vi "init_img_Q.vi"(2 "max queue size (-1, unlimited)":i32) -> (8 "Image Q Out":T1)   [LabVIEW 2023]
uses:
  <vilib>/vision/Image Controls.llb/IMAQ Image.ctl
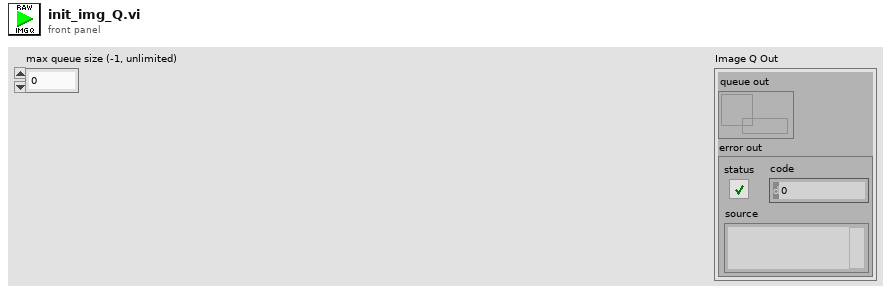
[diagram p1: front panel]
types:
  T1 = cluster{"queue out":refnum<queue>, "error out":errorcluster}
  T2 = typedef "IMAQ Image.ctl" = refnum<image>
  T3 = cluster{"Image Out":T2, "Image Data":cluster{"Actual Width":u32, "Actual Height":u32, "Buffer Number":i32}, "Imaging Variables In":cluster{"Region of interest":i32[], "Number of buffers":u32, "Frame timeout (ms)":u32}}
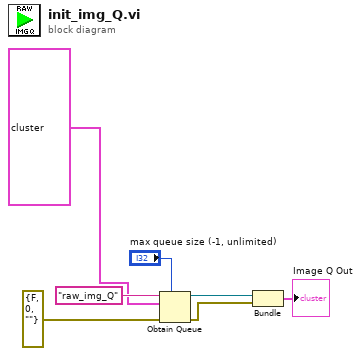
[diagram p0: block diagram]
diagram:
  n1 = Obtain Queue(max queue size (-1, unlimited)="max queue size (-1, unlimited)", name (unnamed)="raw_img_Q", element data type=T3 {"Image Out"=refnum, "Image Data"={"Actual Width"=0, "Actual Height"=0, "Buffer Number"=0}, "Imaging Variables In"={"Region of interest"=[], "Number of buffers"=0, "Frame timeout (ms)"=0}} ("output cluster"), error in (no error)=errorcluster {"status"=FALSE, "code"=0, "source"=""}) -> (queue out=w7:refnum<queue>, error out=w6:errorcluster)  [unwired: 1 in, 1 out]
  n2 = Bundle("queue out"=w7, "error out"=w6) -> (→"Image Q Out":T1)  [unwired: 1 in]
